vi "Szybka_obwiednia.vi"(8 "error in (no error)":errorcluster, 10 "Migawka in":dbl, 11 "Array in":dbl[](array[numeric])) -> (0 "error out":errorcluster, 2 "Migawka out":dbl, 3 "Array out":dbl[](array[numeric]))   [LabVIEW 2013]
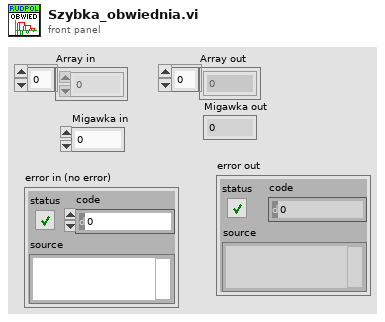
[diagram p1: front panel]
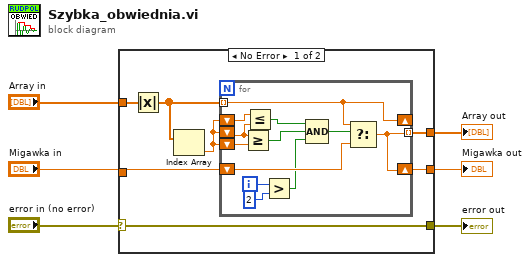
[diagram p0: block diagram]
diagram:
  n1 = case shown="No Error" "error in (no error)" {
    selector: "error in (no error)" -> [w9 w28]
    tunnel: "Array in" -> [w13 w27]
    tunnel: [w10 w27] -> w5
    tunnel: [w9 w28] -> w3
    tunnel: "Migawka in" -> [w8 w26]
    tunnel: [w7 w26] -> w2
    frame No Error {
      n2 = Absolute Value(x=w13) -> (abs(x)=w12:dbl[])
      n3 = Index Array(array=w12) -> (element=w11:dbl)  [unwired: 1 in]
      n4 = for {
        tunnel: w12 -> [w22] mode=indexing
        shift-right: [w22] -> _
        shift-left: w11 -> [w24]
        shift-left: w11 -> [w23]
        shift-left: w11 -> [w25]
        tunnel: [w21] -> w10 mode=indexing
        shift-right: [w21] -> w7
        shift-left: w8 -> [w20]
        i -> [w19]
        n5 = Greater Or Equal?(x=w23, y=w25) -> (x >= y?=w16:bool)
        n6 = Less Or Equal?(x=w24, y=w23) -> (x <= y?=w17:bool)
        n7 = Greater?(x=w19, y=2) -> (0:w15:bool)
        n8 = Compound Arithmetic op=AND(w17, w16, w15) -> (w14:bool)
        n9 = Select(t=w22, s=w14, f=w20) -> (s? t:f=w21:dbl)
      }
    }
    frame Error {
    }
  }
  "Array out" <- w5
  "error out" <- w3
  "Migawka out" <- w2
